vi "VI Interpreter.vi"(8 "error in":errorcluster, 11 "vi reference":refnum<vi>) -> (0 "error out":errorcluster, 3 "VI Interpreter out":refnum<class "VI Interpreter.lvclass">)   [LabVIEW 2014, in "VI Interpreter.lvclass"]
uses:
  VI Interpreter.lvclass
  VI Interpreter.lvclass/VI Interpreter.ctl
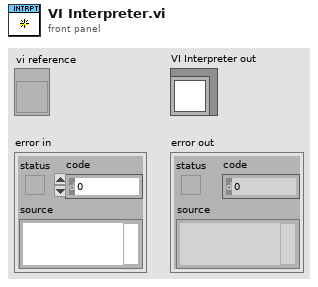
[diagram p1: front panel]
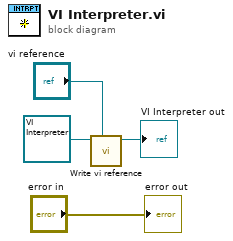
[diagram p0: block diagram]
diagram:
  n1 = call "Write vi reference.vi"("vi reference"="vi reference", "VI Interpreter in"=refnum<class "VI Interpreter.lvclass"> refnum) -> ("VI Interpreter out"=→"VI Interpreter out":refnum<class "VI Interpreter.lvclass">)  [unwired: 7 in]
  "error out" <- "error in"
